vi "From CSV File.vi"(8 "error in (no error)":errorcluster, 9 "Path":path, 10 "engine in":refnum<class "engine configuration.lvclass">, 11 "J1939 editor node in":refnum<class "J1939 editor node.lvclass">) -> (0 "error out":errorcluster, 1 "Update":bool, 2 "engine out":refnum<class "engine configuration.lvclass">, 3 "J1939 editor node out":refnum<class "J1939 editor node.lvclass">)   [LabVIEW 2017, in "J1939 editor node.lvclass"]
uses:
  J1939 editor node.lvclass
  <vilib>/NI/Module Execution Interface/Engine Configuration/engine configuration.lvclass
  module/configuration/J1939 configuration.lvclass
  C:/Program Files (x86)/National Instruments/LabVIEW 2017/vi.lib/NI/Configuration Framework/serializable configuration/NISE_CEF_serializable configuration.lvclass
  <vilib>/NI/Configuration Framework/serializable configuration/NISE_CEF_serializable configuration.lvclass/NISE_CEF_serializable configuration.ctl
  module/configuration/J1939 configuration.lvclass/J1939 configuration.ctl
  <vilib>/Utility/file.llb/Read Delimited Spreadsheet (string).vi
  <vilib>/Utility/LVClass/Get LV Class Name.vi
  <vilib>/NI/Configuration Framework/error generator/NISE_error generator.vi
  <vilib>/NI/Tag Bus Module Framework/channel/TBM channel.lvclass
  <vilib>/NI/Configuration Framework/serializable configuration/NISE_CEF_serializable configuration.lvclass
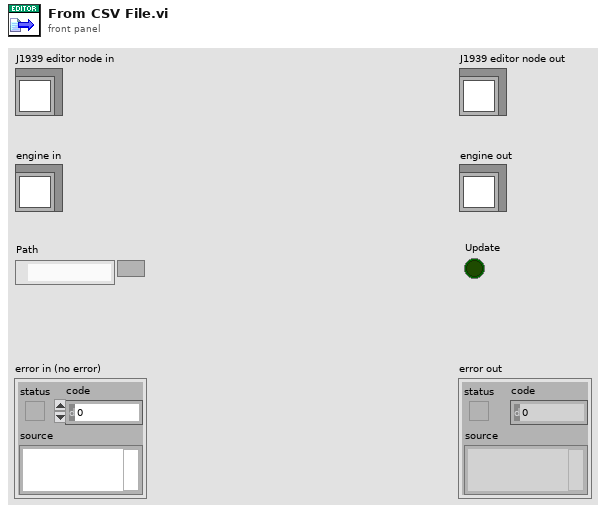
[diagram p1: front panel]
types:
  T1 = typedef "J1939 configuration.lvclass/Line.ctl" = cluster{"channel":refnum<class "TBM channel.lvclass">, "XNET Signal":refnum<k21>}
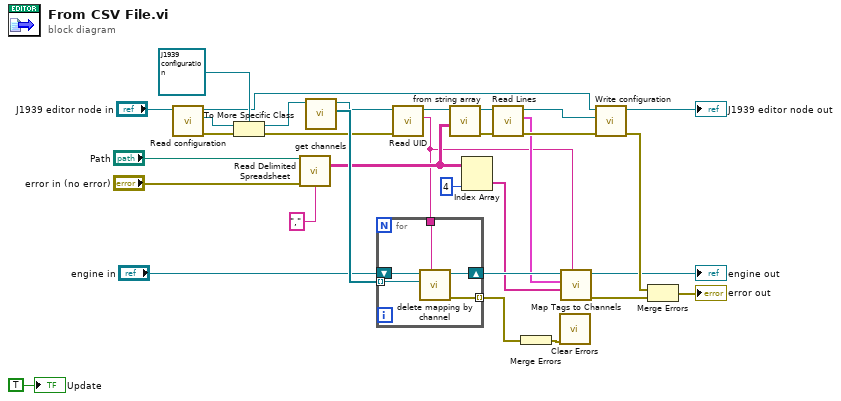
[diagram p0: block diagram]
diagram:
  n1 = call-dynamic "Read configuration.vi"("J1939 editor node in"="J1939 editor node in") -> ("error out"=w28:errorcluster, "configuration"=w26:refnum<class "NISE_CEF_serializable configuration.lvclass">, "J1939 editor node out"=w14:refnum<class "J1939 editor node.lvclass">)  [unwired: 8 in]
  n2 = To More Specific Class(target class=refnum<class "J1939 configuration.lvclass"> refnum ("J1939 configuration"), reference=w26, error in=w28) -> (specific class reference=w23:refnum<class "J1939 configuration.lvclass">, error out=w22:errorcluster)
  n3 = call-poly <vilib>:"Read Delimited Spreadsheet.vi"("file path (dialog if empty)"="Path", "error in (no error)"="error in (no error)", "delimiter (\\t)"="," ("delimiter (\\t)")) -> ("all rows"=w7:string[][])  [unwired: 7 in, 5 out]
  n4 = call-dynamic "get channels.vi"("J1939 configuration in"=w23) -> ("channels"=w25:refnum<class "TBM channel.lvclass">[], "J1939 configuration out"=w24:refnum<class "J1939 configuration.lvclass">)  [unwired: 9 in]
  n5 = call <vilib>:"Read UID.vi"("error in"=w22, "configuration in"=w24) -> ("instance id"=w2:string, "configuration out"=w18:refnum<class "J1939 configuration.lvclass">)  [unwired: 7 in, 1 out]
  n6 = for {
    tunnel: w25 -> [w37] mode=indexing
    tunnel: w2 -> [w36]
    tunnel: [w35] -> w21 mode=indexing
    shift-right: [w33] -> w5
    shift-left: "engine in" -> [w34]
    n7 = call <vilib>:"delete mapping by channel.vi"("owner ID"=w36, "channel"=w37, "engine configuration in"=w34) -> ("error out"=w35:errorcluster, "engine configuration out"=w33:refnum<class "engine configuration.lvclass">)  [unwired: 7 in]
  }
  n8 = call-dynamic "from string array.vi"("String Array"=w7, "module configuration in"=w18) -> ("error out"=w16:errorcluster, "module configuration out"=w17:refnum<class "J1939 configuration.lvclass">)  [unwired: 8 in]
  n9 = Index Array(array=w7, index (col)=4 ("disabled index (col)")) -> (element=w3:string[])  [unwired: 1 in]
  n10 = call "Read Lines.vi"("error in (no error)"=w16, "J1939 configuration in"=w17) -> ("error out"=w13:errorcluster, "Lines"=w4:T1[], "J1939 configuration out"=w15:refnum<class "J1939 configuration.lvclass">)  [unwired: 7 in]
  n11 = Merge Errors(w21) -> (w20:errorcluster)
  n12 = call <vilib>:"Clear Errors.vi"("error in (no error)"=w20) -> ()  [unwired: 5 in, 2 out]
  n13 = call "Map Tags to Channels.vi"("instance id"=w2, "String Array"=w3, "Lines"=w4, "engine configuration in"=w5) -> ("error out"=w1:errorcluster, "engine configuration out"=→"engine out":refnum<class "engine configuration.lvclass">)  [unwired: 6 in]
  n14 = call-dynamic "Write configuration.vi"("error in"=w13, "configuration"=w15, "J1939 editor node in"=w14) -> ("error out"=w12:errorcluster, "J1939 editor node out"=→"J1939 editor node out":refnum<class "J1939 editor node.lvclass">)  [unwired: 7 in]
  n15 = Merge Errors(w12, w1) -> (→"error out":errorcluster)
  "Update" <- TRUE ("Update")
